vi "BuildConstructor.vi"(7 "PythonConverter_BD in":refnum<class "PyConvBD.lvclass">, 8 "error in":errorcluster, 11 "Function in":refnum<class "Function.lvclass">) -> (0 "error out":errorcluster, 3 "Function out":refnum<class "Function.lvclass">, 4 "constructor":string, 5 "PythonConverter_BD out":refnum<class "PyConvBD.lvclass">)   [LabVIEW 2014, in "Function.lvclass"]
uses:
  Function.lvclass
  Python/PythonConverter_BD/PyConvBD.lvclass
  Python/Parsing/Classes/PythonFunction/PythonFunction.lvclass/PythonFunction.ctl
  Python/Parsing/Classes/PythonFunction/PythonFunction.lvclass
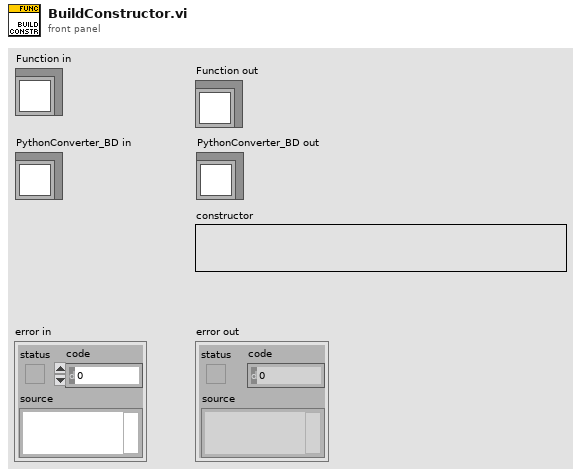
[diagram p1: front panel]
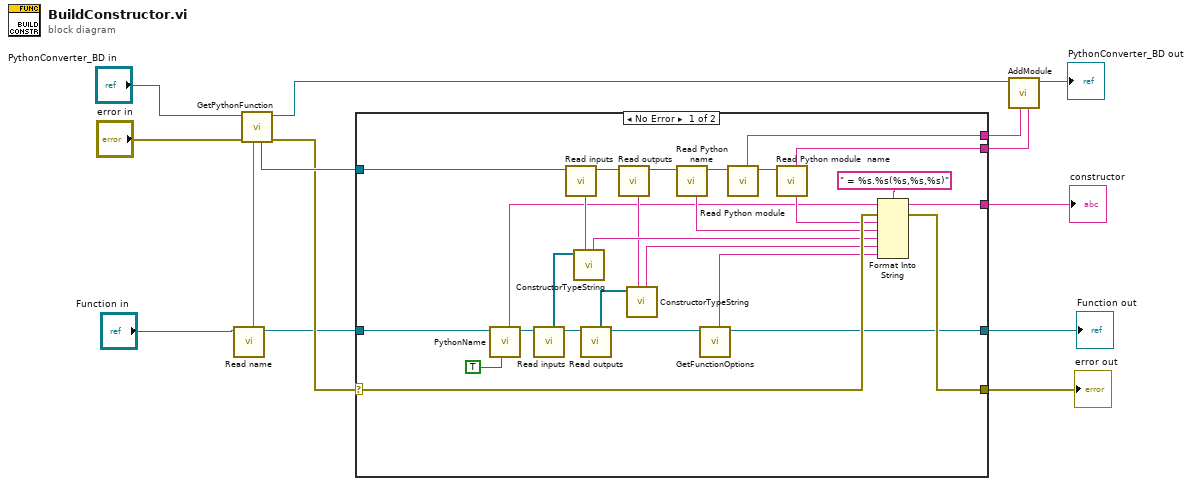
[diagram p0: block diagram]
diagram:
  n1 = call-dynamic "Read name.vi"("Node in"="Function in") -> ("Node out"=w2:refnum<class "Function.lvclass">, "name"=w3:string)  [unwired: 7 in]
  n2 = call "GetPythonFunction.vi"("function name"=w3, "error in"="error in", "PythonConverter_BD in"="PythonConverter_BD in") -> ("error out"=w10:errorcluster, "PythonConverter_BD out"=w8:refnum<class "PyConvBD.lvclass">, "Python function"=w11:refnum<class "PythonFunction.lvclass">)  [unwired: 4 in]
  n3 = case shown="No Error" w10 {
    selector: w10 -> [w40 w42]
    tunnel: [w35 w42] -> w14
    tunnel: [w34 _] -> w13
    tunnel: w2 -> [w24 w41]
    tunnel: w11 -> [w25 _]
    tunnel: [w33 _] -> w7
    tunnel: [w32 _] -> w6
    tunnel: [w16 w41] -> w1
    frame No Error {
      n4 = call-dynamic "PythonName.vi"("add self"=TRUE, "Node in"=w24) -> ("Node out"=w23:refnum<class "Function.lvclass">, "name"=w19:string)  [unwired: 6 in, 2 out]
      n5 = call-dynamic "Read inputs.vi"("Node in"=w23) -> ("Node out"=w21:refnum<class "Function.lvclass">, "inputs"=w22:refnum<class "Terminal.lvclass">[])  [unwired: 7 in]
      n6 = call "Read inputs.vi"("PythonFunction in"=w25) -> ("PythonFunction out"=w26:refnum<class "PythonFunction.lvclass">, "inputs"=w27:string)  [unwired: 7 in]
      n7 = call "ConstructorTypeString.vi"("list"=w27, "terminals"=w22) -> ("constructor string"=w38:string)  [unwired: 7 in]
      n8 = call-dynamic "Read outputs.vi"("Node in"=w21) -> ("Node out"=w17:refnum<class "Function.lvclass">, "outputs"=w20:refnum<class "Terminal.lvclass">[])  [unwired: 7 in]
      n9 = call "Read outputs.vi"("PythonFunction in"=w26) -> ("PythonFunction out"=w28:refnum<class "PythonFunction.lvclass">, "outputs"=w29:string)  [unwired: 7 in]
      n10 = call "ConstructorTypeString.vi"("list"=w29, "terminals"=w20) -> ("constructor string"=w37:string)  [unwired: 7 in]
      n11 = call "Read Python name.vi"("PythonFunction in"=w28) -> ("PythonFunction out"=w31:refnum<class "PythonFunction.lvclass">, "Python name"=w39:string)  [unwired: 7 in]
      n12 = call "GetFunctionOptions.vi"("Function in"=w17) -> ("Function out"=w16:refnum<class "Function.lvclass">, "options"=w15:string)  [unwired: 7 in]
      n13 = call "Read Python module.vi"("PythonFunction in"=w31) -> ("PythonFunction out"=w30:refnum<class "PythonFunction.lvclass">, "Python module"=w33:string)  [unwired: 7 in]
      n14 = call "Read Python module  name.vi"("PythonFunction in"=w30) -> ("Python module  name"=w32:string)  [unwired: 7 in, 1 out]
      n15 = Format Into String(format string=" = %s.%s(%s,%s,%s)", initial string=w19, error in=w40, w32, w39, w38, w37, w15) -> (resulting string=w34:string, error out=w35:errorcluster)
    }
    frame Error {
    }
  }
  "error out" <- w14
  "Function out" <- w1
  "constructor" <- w13
  n16 = call "AddModule.vi"("python module name"=w6, "python module"=w7, "PythonConverter_BD in"=w8) -> ("PythonConverter_BD out"=→"PythonConverter_BD out":refnum<class "PyConvBD.lvclass">)  [unwired: 5 in, 1 out]
